vi "TEST_bench_FXP_L_ye_Bend_u_singleAxis.vi"(6 "NS":u8=9, 8 "Ldist":fxp<+/-,32,5>[](array[numeric])=[0.0, 0.0, 0.0, 0.0, 0.0, 0.0, 0.0, 0.0, 0.0, 0.0, 0.0, 0.0, 0.0, 0.0, 0.0, 0.0, 0.0, 0.0, 0.0, 0.0, 0.0, 0.0, 0.0, 0.0, 0.0, 0.0, 0.0, 0.0, 0.0, 0.0, 0.0, 0.0, 0.0, 0.0, 0.0, 0.0, 0.0, 0.0, 0.0, 0.0, 0.0, 0.0, 0.0, 0.0, 0.0, 0.0, 0.0, 0.0, 0.0, 0.0], 11 "x":fxp<+/-,32,5>[](array[numeric])=[0.0, 0.0, 0.0, 0.0, 0.0, 0.0, 0.0, 0.0, 0.0, 0.0, 0.0, 0.0, 0.0, 0.0, 0.0, 0.0, 0.0, 0.0, 0.0, 0.0, 0.0, 0.0, 0.0, 0.0, 0.0, 0.0, 0.0, 0.0, 0.0, 0.0, 0.0, 0.0, 0.0, 0.0, 0.0, 0.0, 0.0, 0.0, 0.0, 0.0, 0.0, 0.0, 0.0, 0.0, 0.0, 0.0, 0.0, 0.0, 0.0, 0.0]) -> ()   [LabVIEW 2017]
uses:
  fpga_subVIs_ssxy/fixed-point-ss/typeDefs/Lz_bram.ctl
  fpga_subVIs_ssxy/fixed-point-ss/typeDefs/x_vec_bram.ctl
  fpga_subVIs_ssxy/fixed-point-ss/typeDefs/Bz_bram.ctl
  <vilib>/rvi/DataTransferAndStorage/Container/Common/niFpgaContainerExecOnDevCompGetState.vi
  <vilib>/rvi/Emulation/niFpgaEmulationIsFPGAContextNoSignature.vi
  <vilib>/rvi/DataTransferAndStorage/Container/Common/niFpgaContainerGetUniqueNameForEmu.vi
  <vilib>/rvi/Emulation/niFpgaProcessEmulError.vi
  <vilib>/rvi/Emulation/niFpgaSctlEmulationGetInTimedLoop.vi
  <vilib>/rvi/errors/nirviReportUnexpectedCaseInternalError (U32).vi
  <vilib>/rvi/Memory/Memory_Emulation/niFpgaMemoryEmulationCacheClearOnFirstRun.vi
  <vilib>/rvi/Memory/Memory_Emulation/nirvimemoryEmulationManagerCache_MakeExclusive.vi
  <vilib>/rvi/Memory/Memory_Emulation/niFpgaMemoryEmulationValidateCache.vi
  <vilib>/rvi/Memory/Memory_Emulation/nirvimemoryEmulationManagerCache_InsertValue.vi
  <vilib>/Utility/error.llb/Clear Errors.vi
  <vilib>/rvi/Memory/Memory_Emulation/nirvimemoryEmulationManagerCache_ReleaseExclusive.vi
  <vilib>/rvi/Memory/Memory_Emulation/nirvimemoryEmulationManagerCache_GetValue.vi
  <vilib>/rvi/Memory/Memory_Emulation/nirvimemoryEmulationManagerCache_SetValue.vi
  <vilib>/rvi/Emulation/niFpgaSctlEmulationResourceMgr.vi
  <vilib>/rvi/DataTransferAndStorage/Container/XNode/niFpgaContainer.xnode
  <vilib>/rvi/Memory/Memory_Emulation/niFpgaMemoryEmulationRefIn.vi
panel:
  out "xk_1_2":fxp<+/-,32,5>[](array[numeric])
  out "xk_1_1":fxp<+/-,32,5>[](array[numeric])
  in  "U(k): ux":fxp<+/-,18,5>
  in  "y(k)":fxp<+/-,18,5>
  out "yd_est":fxp<+/-,32,5>
  in  "Bz":fxp<+/-,32,5>[](array[numeric])=[0.0, 0.0, 0.0, 0.0, 0.0, 0.0, 0.0, 0.0, 0.0, 0.0, 0.0, 0.0, 0.0, 0.0, 0.0, 0.0, 0.0, 0.0, 0.0, 0.0, 0.0, 0.0, 0.0, 0.0, 0.0, 0.0, 0.0, 0.0, 0.0, 0.0, 0.0, 0.0, 0.0, 0.0, 0.0, 0.0, 0.0, 0.0, 0.0, 0.0, 0.0, 0.0, 0.0, 0.0, 0.0, 0.0, 0.0, 0.0, 0.0, 0.0]
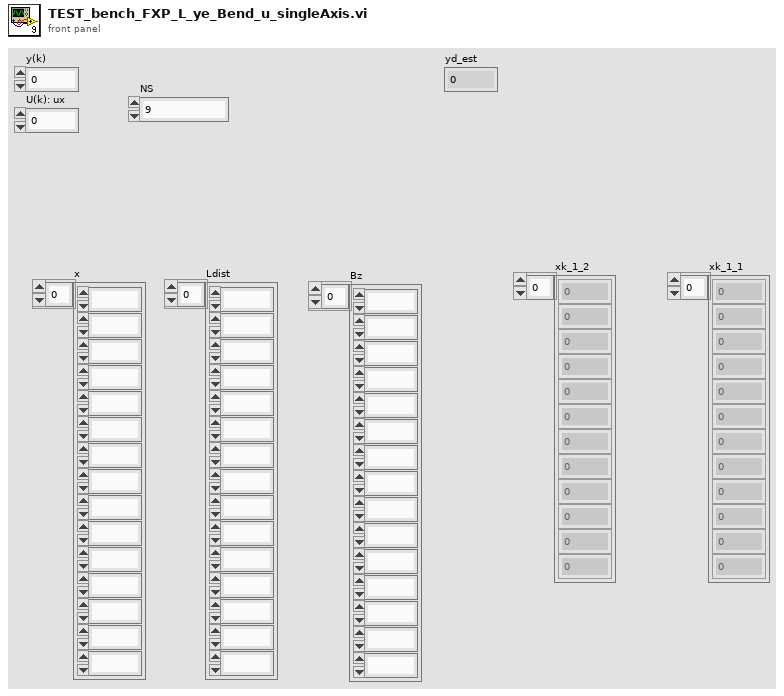
[diagram p1: front panel]
types:
  T1 = typedef "x_vec_bram.ctl" = refnum<k21>
  T2 = typedef "Bz_bram.ctl" = refnum<k21>
  T3 = typedef "Lz_bram.ctl" = refnum<k21>
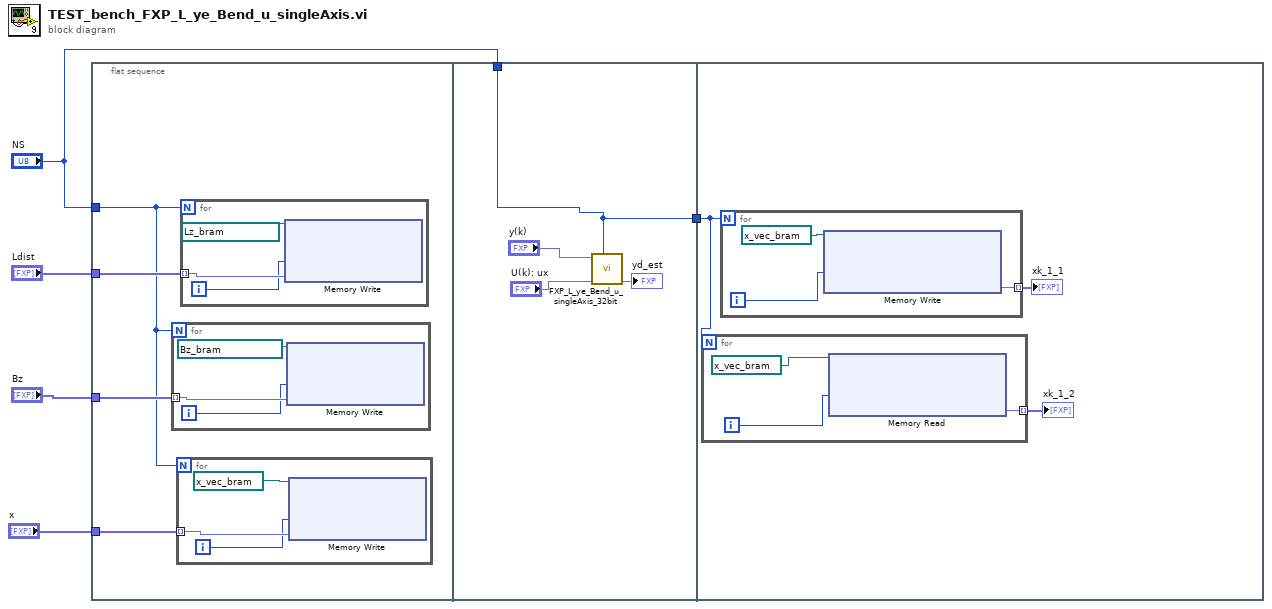
[diagram p0: block diagram]
diagram:
  n1 = flat-sequence {
    tunnel: "NS" -> [w6]
    tunnel: "Ldist" -> [w9]
    tunnel: "x" -> [w8]
    tunnel: "Bz" -> [w7]
    tunnel: "NS" -> [w19]
    tunnel: [w19] -> w1
    tunnel: w1 -> [w23]
    frame #0 {
      n2 = for {
        N: w6 -> [_]
        tunnel: w7 -> [w15] mode=indexing
        i -> [w14]
        n3 = xnode "Memory Write"("Address"=w14, "Data"=w15, "Memory In"=T2 "Bz_FXP_col1" ("Memory")) -> ()  [unwired: 1 out]
      }
      n4 = for {
        N: w6 -> [_]
        tunnel: w8 -> [w12] mode=indexing
        i -> [w11]
        n5 = xnode "Memory Write"("Address"=w11, "Data"=w12, "Memory In"=T1 "xk_1_0" ("Memory")) -> ()  [unwired: 1 out]
      }
      n6 = for {
        N: w6 -> [_]
        tunnel: w9 -> [w18] mode=indexing
        i -> [w17]
        n7 = xnode "Memory Write"("Address"=w17, "Data"=w18, "Memory In"=T3 "L_FXP_col1" ("Memory")) -> ()  [unwired: 1 out]
      }
    }
    frame #1 {
      n8 = call "FXP_L_ye_Bend_u_singleAxis_32bit.vi"("NS"=w19, "U(k): ux"="U(k): ux", "Y(k): x"="y(k)") -> ("yd_est"=→"yd_est":fxp<+/-,32,5>)  [unwired: 7 in, 1 out]
    }
    frame #2 {
      n9 = for {
        N: w23 -> [_]
        tunnel: [w26] -> w24 mode=indexing
        i -> [w27]
        n10 = xnode "Memory Read"("Address"=w27, "Memory In"=T1 "xk_0_2" ("Memory")) -> ("Data"=w26:fxp<+/-,32,6>)  [unwired: 1 out]
      }
      "xk_1_2" <- w24
      n11 = for {
        N: w23 -> [_]
        tunnel: [w30] -> w25 mode=indexing
        i -> [w31]
        n12 = xnode "Memory Write"("Address"=w31, "Memory In"=T1 "xk_0_1" ("Memory")) -> ("Data"=w30:fxp<+/-,32,6>)  [unwired: 1 out]
      }
      "xk_1_1" <- w25
    }
  }
